vi "Basic Averaged DC-RMS.vi"   [LabVIEW 2022 SP3, in "NI_MAPro.lvlib"]
doc: "Calculates the DC and RMS values of an input waveform or array of waveforms. This VI is similar to the Averaged DC-RMS VI, but this VI returns only one <B>DC value</B> and one <B>RMS value</B> per input waveform."
uses:
  NI_MAPro.lvlib
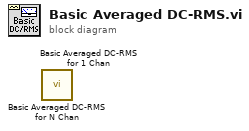
[diagram p0: block diagram]
diagram:
  n1 = call "Basic Averaged DC-RMS for N Chan.vi"() -> ()  [unwired: 8 in, 4 out]
  n2 = call "Basic Averaged DC-RMS for 1 Chan.vi"() -> ()  [unwired: 8 in, 4 out]
